vi "PH_AxisGUI_BaseClass.PC Set Settings.vi"(0 "VI in":refnum<vi>, 2 "Axis":i32=-1, 3 "NewVal":T1 caption="Settings to set", 5 "error in (no error)":errorcluster) -> (14 "VI out":refnum<vi>, 19 "error out":errorcluster)   [LabVIEW 2014, in "PH_AxisGUI_BaseClass.lvlib"]
doc: "This VI acts on an axis."
uses:
  PH_AxisGUI_BaseClass.lvlib
  PH_Stepmotor_BaseClass/PH_Stepmotor_BaseClass.Axis Settings.ctl
  PH_Stepmotor_BaseClass/PH_Stepmotor_BaseClass.Motor Type.ctl
  PH_Stepmotor_BaseClass/PH_Stepmotor_BaseClass.lvlib
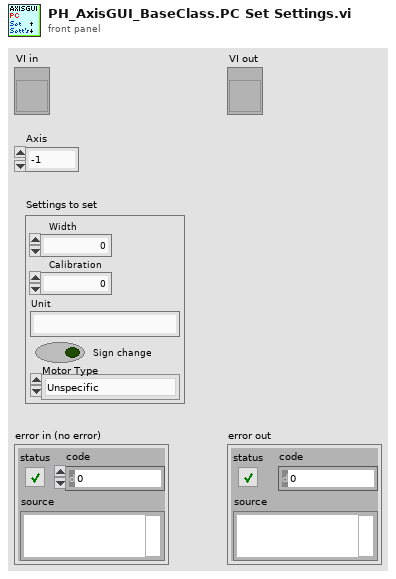
[diagram p1: front panel]
types:
  T1 = typedef "PH_Stepmotor_BaseClass.lvlib/PH_Stepmotor_BaseClass.Axis Settings.ctl" = cluster{"Sign change":bool, "Width":dbl, "Calibration":dbl, "Unit":string, "Motor Type":T2, "Unit Width":string, "Unit CF":string}
  T2 = typedef "PH_Stepmotor_BaseClass.lvlib/PH_Stepmotor_BaseClass.Motor Type.ctl" = enum16{"Unspecific", "OWIS 49.120.2633", "OWIS 49.060.1033", "OWIS 43.040.2558", "Diamond Motion 2200 series", "OWIS 49.120.266B.MV6", "Calorimeter", "Linear Stage 1", "MICOS VT-80", "MICOS VT-80 S", "Standa Rotstage nt0.95A", "PUF RA 320.200", "PUF RA 800.200", "PUF RA 800.400", "PUF RA 400.50", "1324.nn.800.50", "1324.n9c.800.50", "1324.nn.320.200", "1324.nn.400.200", "1324.nn.800.200", "1324.nn.400.50", "1324.8c9c.800.50", "1324.8c9c.400.200"}
  T3 = typedef "PH_Stepmotor_BaseClass.lvlib/PH_Stepmotor_BaseClass.Axis Address.ctl" = cluster{"Instance":string, "Motor Nr":i32}
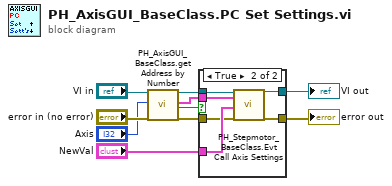
[diagram p0: block diagram]
diagram:
  n1 = call "PH_AxisGUI_BaseClass.get Address by Number.vi"("VI in"="VI in", "Axis"="Axis", "error in (no error)"="error in (no error)") -> ("VI out"=w7:refnum<vi>, "Address"=w3:T3, "Axis exists and is not moving?"=w1:bool, "error out"=w6:errorcluster)  [unwired: 12 in, 1 out]
  n2 = case shown="True" w1 {
    tunnel: "NewVal" -> [_ w18]
    tunnel: [w12 w17] -> w9
    tunnel: [w11 w16] -> w8
    tunnel: w7 -> [w12 w15]
    tunnel: w6 -> [w11 w14]
    tunnel: w3 -> [_ w13]
    frame False {
    }
    frame True {
      n3 = call "PH_Stepmotor_BaseClass.Evt Call Axis Settings.vi"("i ref in"=w15, "Address"=w13, "Settings to set"=w18, "error in"=w14) -> ("i ref out"=w17:refnum<vi>, "error out"=w16:errorcluster)  [unwired: 14 in]
    }
  }
  "VI out" <- w9
  "error out" <- w8
